vi "PCO_RecorderSetAutoExpRegions.vi"(0 "phRec":u64, 1 "wRoiY0Arr":u16[](array[numeric])=array[4097 elements], 5 "phCam":u64, 7 "wRegionType":u16(ring) items=["REGION_TYPE_BALANCED", "REGION_TYPE_CENTER_BASED", "REGION_TYPE_CORNER_BASED", "REGION_TYPE_FULL", "REGION_TYPE_CUSTOM"], 9 "wRoiX0Arr":u16[](array[numeric])=array[4097 elements], 11 "error in (no error)":errorcluster {"code" format="%x"}) -> (4 "phRec out":u64, 6 "ErrorMessage":i32 format="%x", 15 "error out":errorcluster {"code" format="%x"})   [LabVIEW 2019, in "Recorder.lvlib"]
doc: "int WINAPI PCO_RecorderSetAutoExpRegions(HANDLE phRec, HANDLE phCam, WORD regionType, WORD* roiX0Arr, WORD* roiY0Arr, WORD arrLength);"
uses:
  Recorder.lvlib
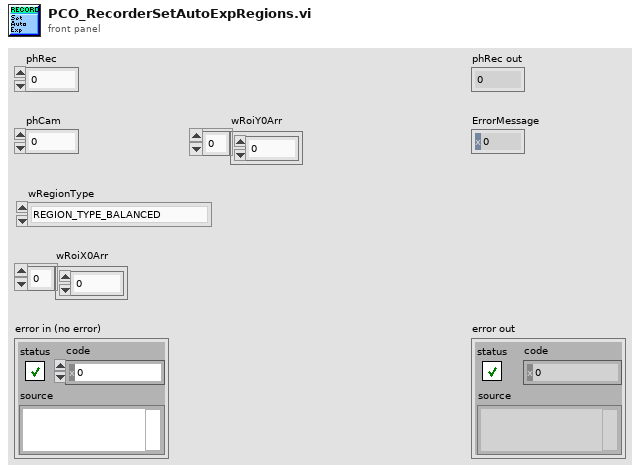
[diagram p1: front panel]
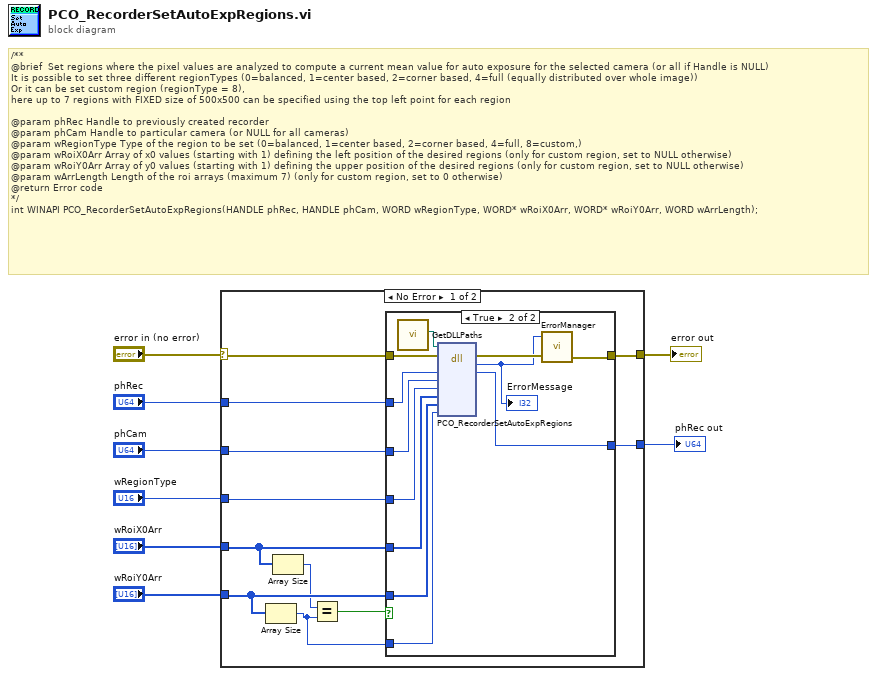
[diagram p0: block diagram]
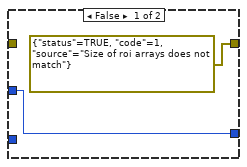
[diagram p2: hidden frame]
diagram:
  # "/**\n@brief  Set regions where the pixel values are analyzed to compute a current mean value for auto exposure for the selected camera (or all if Handle is NULL)\nIt is possible to set three different regionTypes (0=balanced, 1=center based, 2=corner based, 4=full (equally distributed over whole image))\nOr it can be set custom region (regionType = 8),\nhere up to 7 regions with FIXED size of 500x500 can be specified using the top left point for each region\n\n@param phRec Handle to previously created recorder\n@param phCam Handle to particular camera (or NULL for all cameras)\n@param wRegionType Type of the region to be set (0=balanced, 1=center based, 2=corner based, 4=full, 8=custom,)\n@param wRoiX0Arr Array of x0 values (starting with 1) defining the left position of the desired regions (only for custom region, set to NULL otherwise)\n@param wRoiY0Arr Array of y0 values (starting with 1) defining the upper position of the desired regions (only for custom region, set to NULL otherwise)\n@param wArrLength Length of the roi arrays (maximum 7) (only for custom region, set to 0 otherwise)\n@return Error code\n*/\nint WINAPI PCO_RecorderSetAutoExpRegions(HANDLE phRec, HANDLE phCam, WORD wRegionType, WORD* wRoiX0Arr, WORD* wRoiY0Arr, WORD wArrLength);"
  n1 = case shown="No Error" "error in (no error)" {
    selector: "error in (no error)" -> [w14 w34]
    tunnel: "phRec" -> [w19 w35]
    tunnel: [w18 w35] -> w7
    tunnel: "phCam" -> [w17 _]
    tunnel: "wRegionType" -> [w16 _]
    tunnel: "wRoiX0Arr" -> [w11 _]
    tunnel: "wRoiY0Arr" -> [w13 _]
    tunnel: [w15 w34] -> w2
    frame No Error {
      n2 = Array Size(array=w13) -> (size(s)=w9:i32)
      n3 = Array Size(array=w11) -> (size(s)=w12:i32)
      n4 = Equal?(x=w12, y=w9) -> (x = y?=w10:bool)
      n5 = case shown="True" w10 {
        tunnel: w19 -> [w20 w33]
        tunnel: [w20 w32] -> w18
        tunnel: w17 -> [_ w31]
        tunnel: w16 -> [_ w30]
        tunnel: w11 -> [_ w29]
        tunnel: w13 -> [_ w28]
        tunnel: [errorcluster {"status"=TRUE, "code"=1, "source"="Size of roi arrays does not match"} ("error out") w25] -> w15
        tunnel: w14 -> [_ w27]
        tunnel: w9 -> [_ w23]
        frame False {
        }
        frame True {
          n6 = call "GetDLLPaths.vi"() -> ("PCO_Recorder_Path"=w22:path)  [unwired: 9 in, 2 out]
          n7 = dll-call lib="?" fn="PCO_RecorderSetAutoExpRegions"(path in=w22, error in=w27, "phRec"=w33, "phCam"=w31, "wRegionType"=w30, "wRoiX0Arr"=w29, "wRoiY0Arr"=w28, "wArrLength"=w23) -> (error out=w26:errorcluster, "return type"=w24:i32, "phRec"=w32:u64)  [unwired: 6 in, 1 out]
          "ErrorMessage" <- w24
          n8 = call "ErrorManager.vi"("error in (no error)"=w26, "error code"=w24) -> ("error out"=w25:errorcluster)  [unwired: 3 in]
        }
      }
    }
    frame Error {
    }
  }
  "phRec out" <- w7
  "error out" <- w2
